vi "waveform to t-Y cluster.vi"   [LabVIEW 2010, in "common.lvlib"]
uses:
  common.lvlib
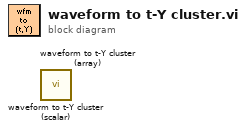
[diagram p0: block diagram]
diagram:
  n1 = call "waveform to t-Y cluster (scalar).vi"() -> ()  [unwired: 1 in, 1 out]
  n2 = call "waveform to t-Y cluster (array).vi"() -> ()  [unwired: 1 in, 1 out]
